vi "VectorToScalar Finger Speed.vi"(9 "error in (no error)":errorcluster, 11 "reference":refnum<k24>) -> (0 "error out":errorcluster, 2 "sqrt(x)":sgl)   [LabVIEW 2014]
uses:
  C:/Users/Frax/Desktop/Progetti avanzati Labview/Smart Wristband/Smart Wristband/Leap Motion VIs 2.0/LeapCSharp.NET4.0.dll
  LeapCSharp.NET4.0.dll
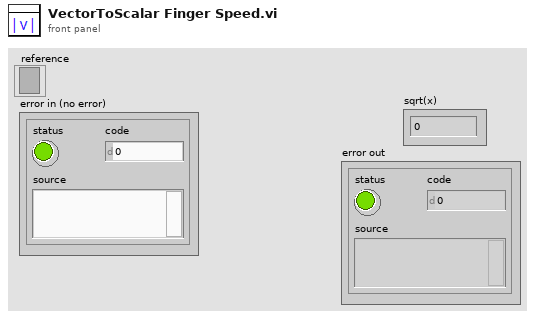
[diagram p1: front panel]
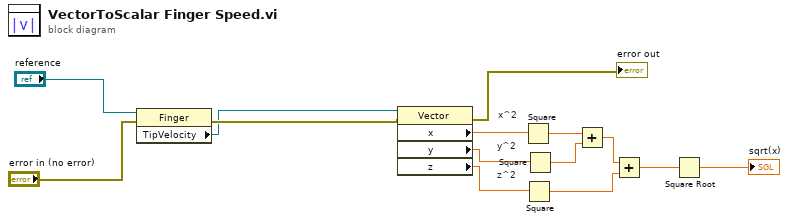
[diagram p0: block diagram]
diagram:
  n1 = property class="Finger"(reference="reference", error in="error in (no error)") -> (error out=w14:errorcluster, "TipVelocity"=w13:refnum<k24>)  [unwired: 1 out]
  n2 = property class="Vector"(reference=w13, error in=w14) -> (error out=→"error out":errorcluster, "x"=w12:sgl, "y"=w11:sgl, "z"=w10:sgl)  [unwired: 1 out]
  n3 = Square "x^2"(x=w12) -> (x^2=w9:sgl)
  n4 = Square "z^2"(x=w10) -> (x^2=w6:sgl)
  n5 = Square "y^2"(x=w11) -> (x^2=w8:sgl)
  n6 = Add(x=w9, y=w8) -> (x+y=w7:sgl)
  n7 = Add(x=w7, y=w6) -> (x+y=w5:sgl)
  n8 = Square Root(x=w5) -> (sqrt(x)=→"sqrt(x)":sgl)
